vi "3-phase RMS.vi"(4 "Vabc":T1) -> (1 "RMS":fxp<+,55,5>)   [LabVIEW 2016]
types:
  T1 = cluster{"A":fxp<+/-,18,4>, "B":fxp<+/-,18,4>, "C":fxp<+/-,18,4>}
  T2 = cluster{"A":fxp<+,35,7>, "B":fxp<+,35,7>, "C":fxp<+,35,7>}
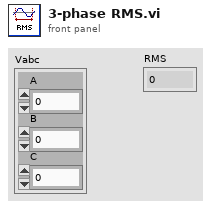
[diagram p1: front panel]
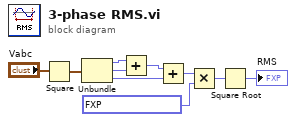
[diagram p0: block diagram]
diagram:
  n1 = Square(x="Vabc") -> (x^2=w10:T2)
  n2 = Unbundle(w10) -> ("A"=w8:fxp<+,35,7>, "B"=w6:fxp<+,35,7>, "C"=w5:fxp<+,35,7>)
  n3 = Add(x=w8, y=w6) -> (x+y=w7:fxp<+,36,8>)
  n4 = Add(x=w7, y=w5) -> (x+y=w4:fxp<+,36,8>)
  n5 = Multiply(x=w4, y=fxp<+,16,1> 0.33331298828125) -> (x*y=w3:fxp<+,52,9>)
  n6 = Square Root(x=w3) -> (sqrt(x)=→"RMS":fxp<+,55,5>)
